vi "DemoUI.vi"() -> ()   [LabVIEW 2020, in "UI_Main.lvclass"]
uses:
  UI_Main_Test/UI_Main.lvclass
  DAQmx.AI/Typedefs/4461AIRange.ctl
  DAQmx.AI/DAQmx.AI.lvclass
panel:
  in  "System Array 2":T1(array[cluster]) {"AO f" min=0.001 max=10000.0; "AO DC" format="%#_6p"; "AO Amp" format="%#_6p"}
  in  "AO f (Hz)":dbl[](array[numeric])=[13.1, 13.0, 13.0, 13.0, 13.0, 13.0, 13.0, 13.0] min=0.001 max=10000.0
  in  "function":T2(array[ring])=[enum."Sine Wave", enum."Sine Wave", enum."Sine Wave", enum."Sine Wave", enum."Sine Wave", enum."Sine Wave", enum."Sine Wave", enum."Sine Wave"]
  in  "AO phi (deg)":dbl[](array[numeric])=[0.0, 0.0, 0.0, 0.0, 0.0, 0.0, 0.0, 0.0]
  in  "AO DC (V)":dbl[](array[numeric])=[0.0, 0.0, 0.0, 0.0, 0.0, 0.0, 0.0, 0.0] format="%#_6p"
  in  "AO amp (V)":dbl[](array[numeric])=[0.01, 0.0, 0.0, 0.0, 0.0, 0.0, 0.0, 0.0] format="%#_6p"
  in  "System Array":T3[](array[typedef])
  # "Amp (V)"
  # "DC (V)"
  # "f (Hz)"
  # "phi (°)"
  # "function"
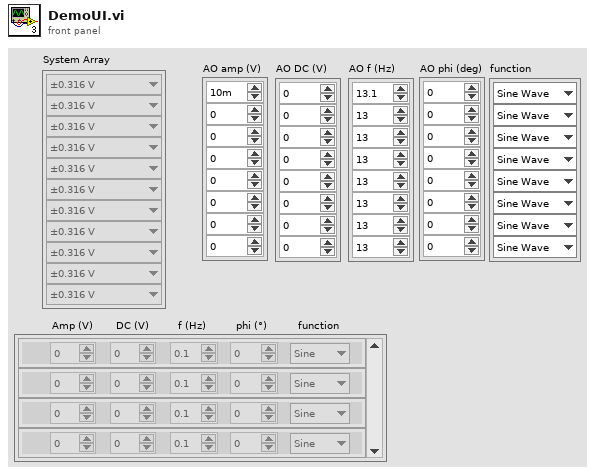
[diagram p1: front panel]
types:
  T1 = cluster{"AO Amp":dbl, "AO DC":dbl, "AO f":dbl, "AO phi":dbl, "Enum":enum16{"Sine", "Triangle", "Square"}}[]
  T2 = enum16{"Sine Wave", "Triangle Wave", "Square Wave", "Sawtooth Wave"}[]
  T3 = typedef "DAQmx.AI.lvclass/4461AIRange.ctl" = enum16{"±0.316 V", "±1.00 V", "±3.16 V", "±10.0 V", "±31.6 V", "±42.4 V"}
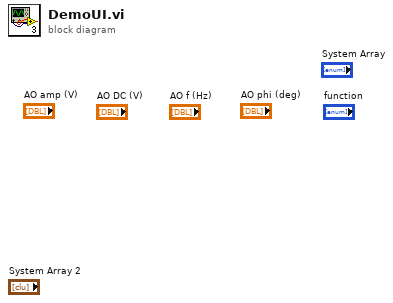
[diagram p0: block diagram]
diagram:
